vi "Path Array to Path String.vi"(11 "path array":string[](array[string])) -> (3 "path":string)   [LabVIEW 2020, in "Variant Data Manipulation.lvlib"]
uses:
  Variant Data Manipulation.lvlib
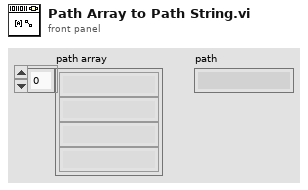
[diagram p1: front panel]
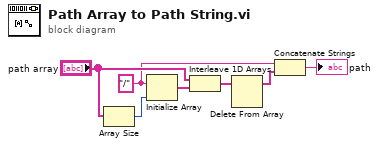
[diagram p0: block diagram]
diagram:
  w3 = "/" ("delimiter (Tab)")
  n1 = Array Size(array="path array") -> (size(s)=w6:i32)
  n2 = Initialize Array(w3, w6) -> (w4:string[])
  n3 = Interleave 1D Arrays("path array", w4) -> (w1:string[])
  n4 = Delete From Array(array=w1) -> (array with subset deleted=w2:string[])  [unwired: 2 in, 1 out]
  n5 = Concatenate Strings(w3, w2) -> (→"path":string)
